vi "Event-Driven State Machine - VI Window Customization.vi"() -> ()   [LabVIEW 2020]
uses:
  support/State Machine Data.ctl
  support/States.ctl
  <vilib>/DAQmx/create/channels.llb/DAQmx Create Channel (AO-Voltage-Basic).vi
  <vilib>/DAQmx/configure/timing.llb/DAQmx Timing (Sample Clock).vi
  <vilib>/DAQmx/read.llb/DAQmx Read (Analog 2D DBL NChan NSamp).vi
  <vilib>/Utility/file.llb/Write Delimited Spreadsheet (DBL).vi
  <vilib>/DAQmx/write.llb/DAQmx Write (Analog DBL 1Chan 1Samp).vi
  <vilib>/DAQmx/create/channels.llb/DAQmx Create Channel (AI-Voltage-Basic).vi
panel:
  out "RMS Results Per Channel":dbl[](array[numeric])
  out "Threshold exceeded?":bool
  in  "Acquire":bool
  in  "Samples per channel":i32=100
  in  "Sample Rate":dbl=1000.0
  in  "AI Voltage Channel":tag="PCI-6221/ai0, PCI-6221/ai2:3"
  in  "AO Voltage Channel":tag="PCI-6221/ao0"
  in  "Generate Stimulus":bool
  in  "Threshold (rms)":dbl=1.0
  in  "Clear":bool
  in  "Exit":bool
  out "Graph":dbl[][](graph)
  # "Analysis"
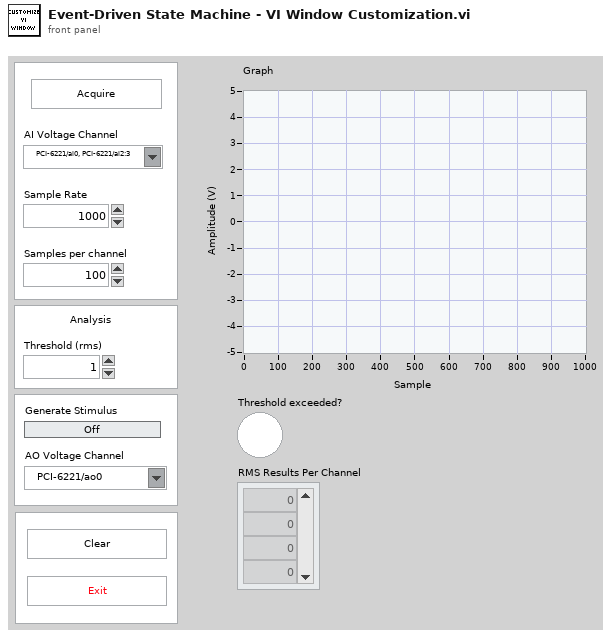
[diagram p1: front panel]
types:
  T1 = typedef "States.ctl" = enum16{"Initialize", "Wait for Event", "Acquire", "Analyze", "Log", "Clear", "Update Stimulus", "Update UI", "Exit"}
  T2 = typedef "State Machine Data.ctl" = cluster{"Acquisition Data":dbl[][], "Stimulus Value":bool}
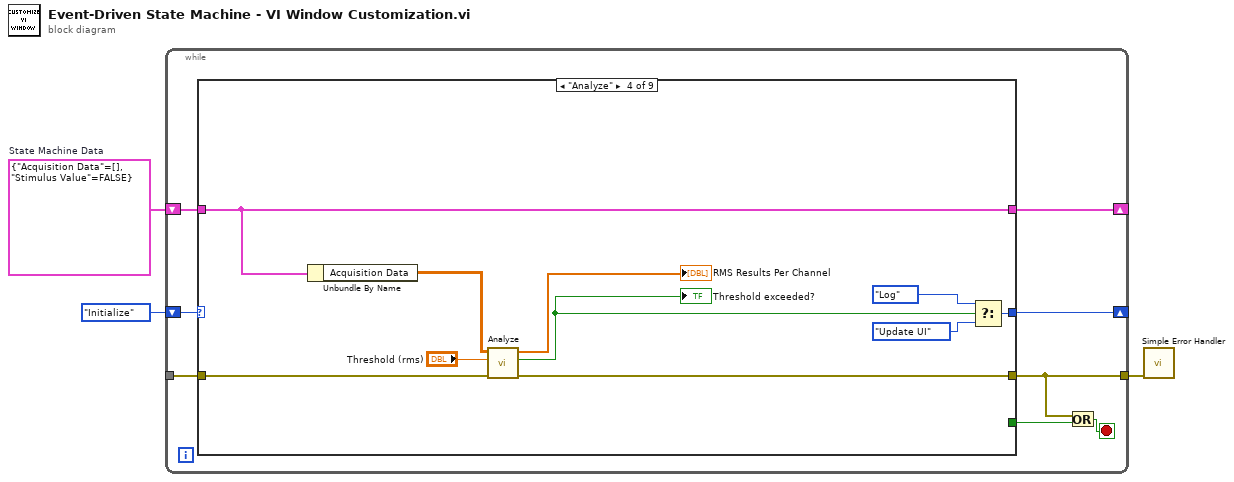
[diagram p0: block diagram]
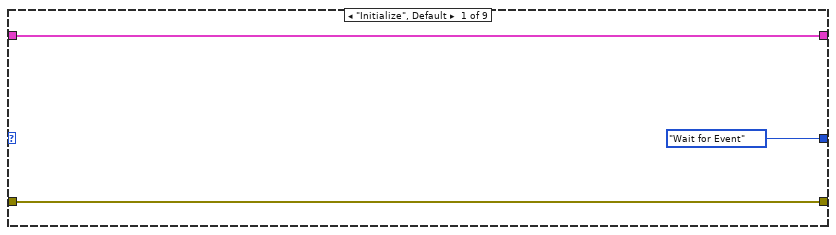
[diagram p2: hidden frame]
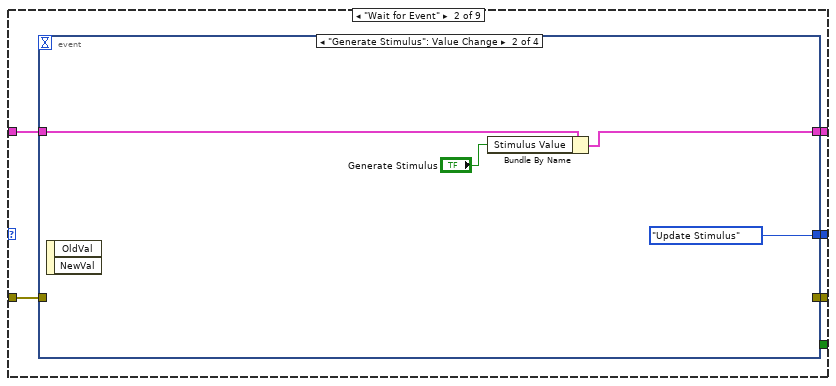
[diagram p3: hidden frame]
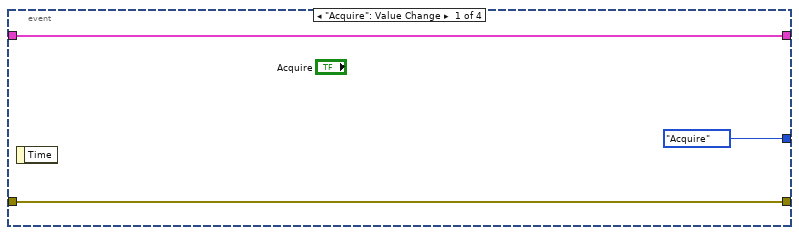
[diagram p4: hidden frame]
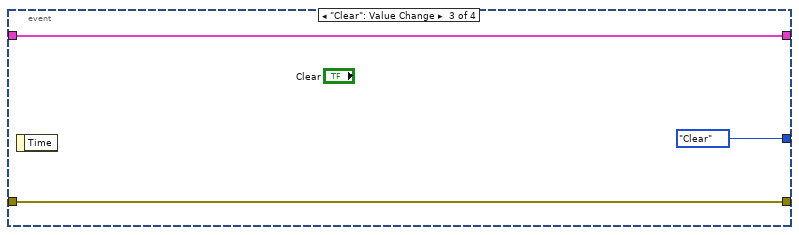
[diagram p5: hidden frame]
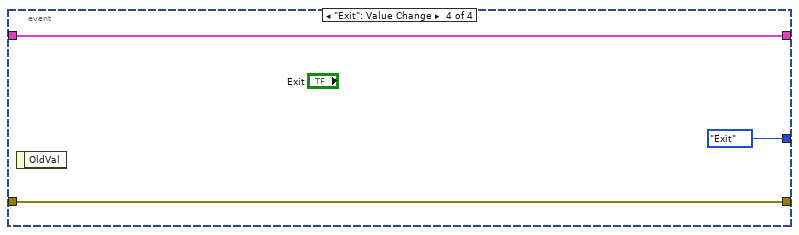
[diagram p6: hidden frame]
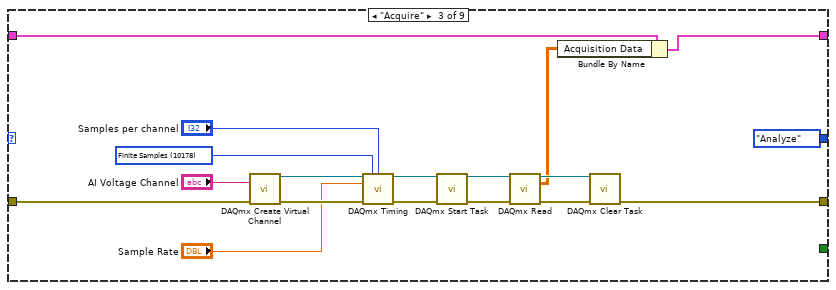
[diagram p7: hidden frame]
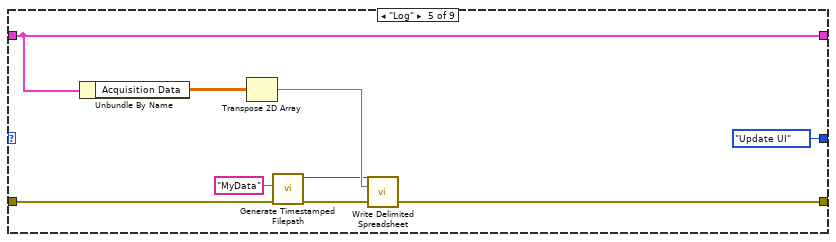
[diagram p8: hidden frame]
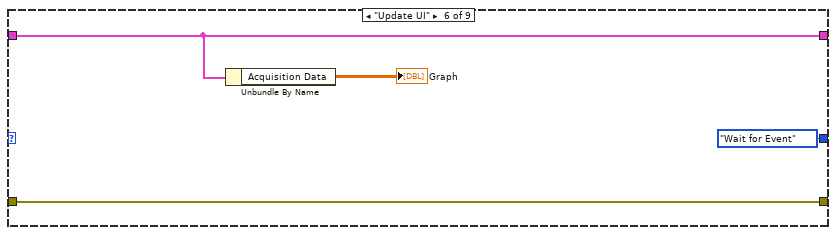
[diagram p9: hidden frame]
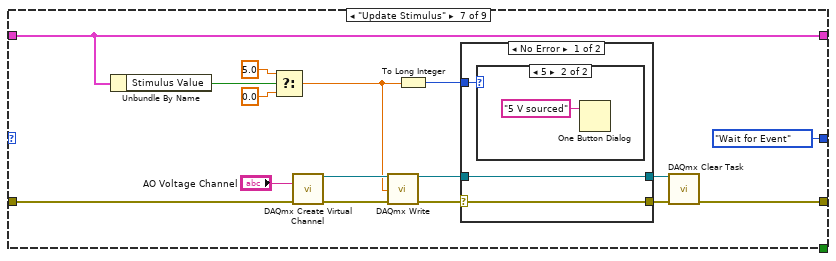
[diagram p10: hidden frame]
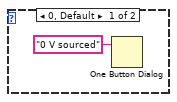
[diagram p11: hidden frame]
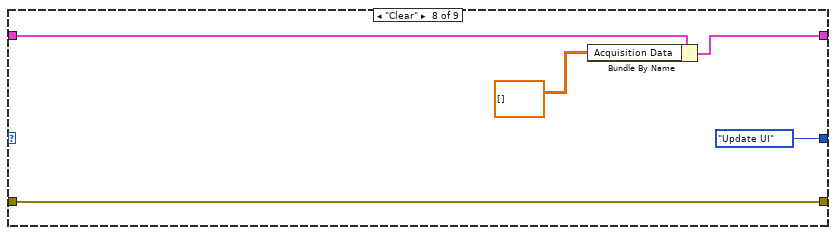
[diagram p13: hidden frame]
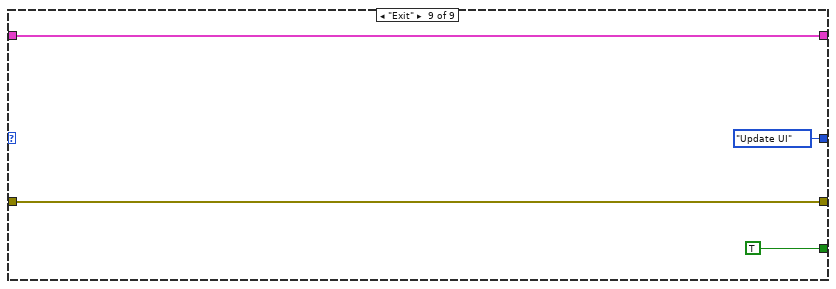
[diagram p14: hidden frame]
diagram:
  w2 = T2 {"Acquisition Data"=[], "Stimulus Value"=FALSE}  # State Machine Data
  n1 = while {
    shift-right: [w8] -> _
    shift-left: States."Initialize" ("States") -> [w11]
    shift-right: [w9] -> _
    shift-left: w2 -> [w10]
    tunnel: [w7] -> _
    tunnel: [w6] -> w1
    stop <- w4 stop-if-true
    n2 = case shown="\"Analyze\"" w11 {
      tunnel: w10 -> [w14 w19 w38 w60 w68 w72 w89 w100 w104]
      tunnel: [w14 w18 w34 w60 w68 w72 w89 w98 w104] -> w9
      tunnel: [States."Wait for Event" ("States") w15 States."Analyze" ("States") w52 States."Update UI" ("States") States."Wait for Event" ("States") States."Wait for Event" ("States") States."Update UI" ("States") States."Update UI" ("States")] -> w8
      tunnel: [w12 w17 w50 w57 w66 w73 w83 w101 w105] -> w7
      tunnel: [w12 w16 w36 w55 w62 w73 w84 w101 w105] -> w6
      tunnel: [_ _ _ _ _ _ _ _ TRUE] -> w5
      frame "Initialize", Default {
      }
      frame "Wait for Event" {
        n3 = event shown="[1] \"Generate Stimulus\": Value Change" {
          selector: _ -> [_ _ _ _]
          dyn-events: _ -> [_ _ _ _]
          timeout: _ -> [_ _ _ _]
          tunnel: w19 -> [w21 w26 w29 w31]
          tunnel: [w21 w25 w29 w31] -> w18
          tunnel: w17 -> [w22 _ w28 w32]
          tunnel: [w22 _ w28 w32] -> w16
          tunnel: [States."Acquire" ("Enum") States."Update Stimulus" ("Enum") States."Clear" ("Enum") States."Exit" ("Enum")] -> w15
          event "Acquire": Value Change {
            n4 = event-data() -> ()  [unwired: 1 in, 1 out]
          }
          event "Generate Stimulus": Value Change {
            n5 = event-data() -> ()  [unwired: 1 in, 2 out]
            n6 = Bundle By Name(cluster=w26, "Stimulus Value"="Generate Stimulus") -> (w25:T2)
          }
          event "Clear": Value Change {
            n7 = event-data() -> ()  [unwired: 1 in, 1 out]
          }
          event "Exit": Value Change {
            n8 = event-data() -> ()  [unwired: 1 in, 1 out]
          }
        }
      }
      frame "Acquire" {
        w46 = 10178 items=["Finite Samples"=10178, "Continuous Samples"=10123, "Hardware Timed Single Point"=12522] ("sample mode")
        n9 = call-poly <vilib>:"DAQmx Create Virtual Channel.vi"("physical channels"="AI Voltage Channel", "error in"=w50) -> ("task out"=w47:refnum<k21>, "error out"=w48:errorcluster)  [unwired: 12 in]
        n10 = call-poly <vilib>:"DAQmx Timing.vi"("task/channels in"=w47, "sample mode"=w46, "samples per channel"="Samples per channel", "rate"="Sample Rate", "error in"=w48) -> ("task out"=w44:refnum<k21>, "error out"=w43:errorcluster)  [unwired: 9 in]
        n11 = call <vilib>:"DAQmx Start Task.vi"("task/channels in"=w44, "error in"=w43) -> ("task out"=w42:refnum<k21>, "error out"=w41:errorcluster)  [unwired: 12 in]
        n12 = call-poly <vilib>:"DAQmx Read.vi"("task/channels in"=w42, "error in"=w41) -> ("task out"=w40:refnum<k21>, "data"=w37:dbl[][], "error out"=w39:errorcluster)  [unwired: 11 in]
        n13 = Bundle By Name(cluster=w38, "Acquisition Data"=w37) -> (w34:T2)
        n14 = call <vilib>:"DAQmx Clear Task.vi"("task in"=w40, "error in"=w39) -> ("error out"=w36:errorcluster)  [unwired: 13 in]
      }
      frame "Analyze" {
        n15 = Unbundle By Name(w60) -> ("Acquisition Data"=w59:dbl[][])
        n16 = call "Analyze.vi"("error in (no error)"=w57, "Threshold (rms)"="Threshold (rms)", "N-Channel Data (2D DBL)"=w59) -> ("error out"=w55:errorcluster, "Threshold Exceeded?"=w51:bool, "N-Channel RMS Results"=→"RMS Results Per Channel":dbl[])  [unwired: 5 in, 1 out]
        "Threshold exceeded?" <- w51
        n17 = Select(t=States."Log" ("States"), s=w51, f=States."Update UI" ("States")) -> (s? t:f=w52:T1)
      }
      frame "Log" {
        n18 = Unbundle By Name(w68) -> ("Acquisition Data"=w69:dbl[][])
        n19 = Transpose 2D Array(2D array=w69) -> (transposed array=w65:dbl[][])
        n20 = call "Generate Timestamped Filepath.vi"("Error In"=w66, "appended filename"="MyData") -> ("Error Out"=w63:errorcluster, "timestamped relative filepath"=w64:path)  [unwired: 8 in]
        n21 = call-poly <vilib>:"Write Delimited Spreadsheet.vi"("file path (dialog if empty)"=w64, "2D data"=w65, "error in (no error)"=w63) -> ("error out"=w62:errorcluster)  [unwired: 11 in, 1 out]
      }
      frame "Update UI" {
        n22 = Unbundle By Name(w72) -> ("Acquisition Data"=→"Graph":dbl[][])
      }
      frame "Update Stimulus" {
        n23 = Unbundle By Name(w89) -> ("Stimulus Value"=w80:bool)
        n24 = Select(t=5.0, s=w80, f=0.0) -> (s? t:f=w79:dbl)
        n25 = call-poly <vilib>:"DAQmx Create Virtual Channel.vi"("physical channels"="AO Voltage Channel", "error in"=w83) -> ("task out"=w86:refnum<k21>, "error out"=w85:errorcluster)  [unwired: 12 in]
        n26 = call-poly <vilib>:"DAQmx Write.vi"("task/channels in"=w86, "data"=w79, "error in"=w85) -> ("task out"=w76:refnum<k21>, "error out"=w77:errorcluster)  [unwired: 10 in, 1 out]
        n27 = To Long Integer(number=w79) -> (32bit integer=w78:i32)
        n28 = case shown="No Error" w77 {
          selector: w77 -> [w90 w95]
          tunnel: w78 -> [w92 _]
          tunnel: w76 -> [w91 w96]
          tunnel: [w91 w96] -> w75
          tunnel: [w90 w95] -> w74
          frame No Error {
            n29 = case shown="5" w92 {
              frame 0, Default {
                n30 = One Button Dialog(message="0 V sourced") -> ()  [unwired: 1 in, 1 out]
              }
              frame 5 {
                n31 = One Button Dialog(message="5 V sourced") -> ()  [unwired: 1 in, 1 out]
              }
            }
          }
          frame Error {
          }
        }
        n32 = call <vilib>:"DAQmx Clear Task.vi"("task in"=w75, "error in"=w74) -> ("error out"=w84:errorcluster)  [unwired: 13 in]
      }
      frame "Clear" {
        n33 = Bundle By Name(cluster=w100, "Acquisition Data"=dbl[][] []) -> (w98:T2)
      }
      frame "Exit" {
      }
    }
    n34 = Or(x=w6, y=w5) -> (x .or. y?=w4:bool)
  }
  n35 = call <vilib>:"Simple Error Handler.vi"("error in (no error)"=w1) -> ()  [unwired: 4 in, 5 out]
